vi "To Pretty String (Object).vi"(6 "pretty print? (T)":bool=TRUE, 7 "enable LabVIEW extensions? (T)":bool=TRUE, 8 "error in (no error)":errorcluster, 11 "JSON Value in":refnum<class "JSON Value.lvclass">) -> (0 "error out":errorcluster, 3 "Pretty Print String":string)   [LabVIEW 2016, in "JSON Value.lvclass"]
doc: "Pretty prints the given JSON data in an easier to read format."
uses:
  JSON Value.lvclass
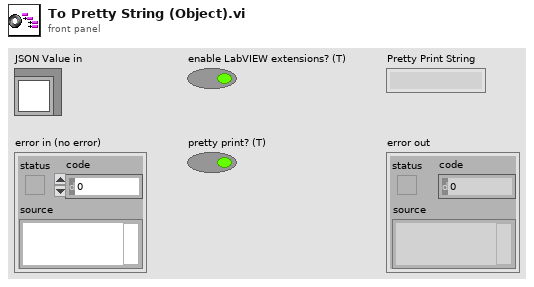
[diagram p1: front panel]
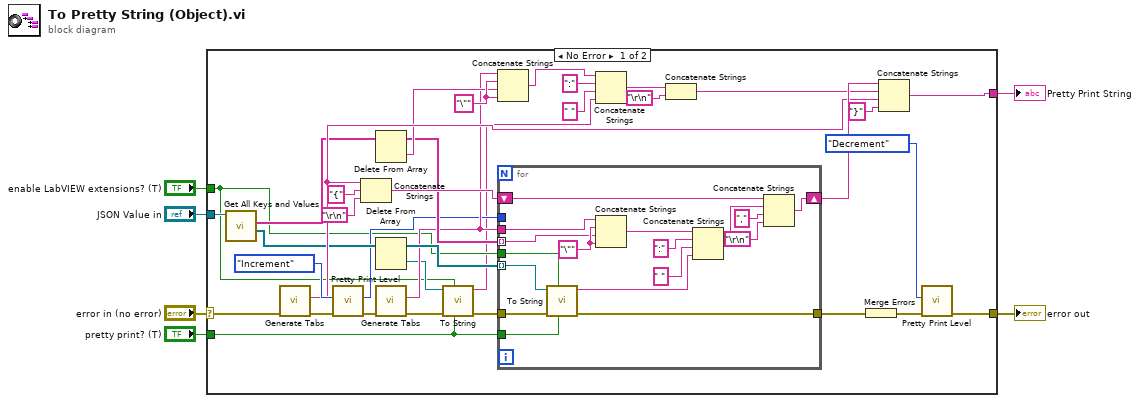
[diagram p0: block diagram]
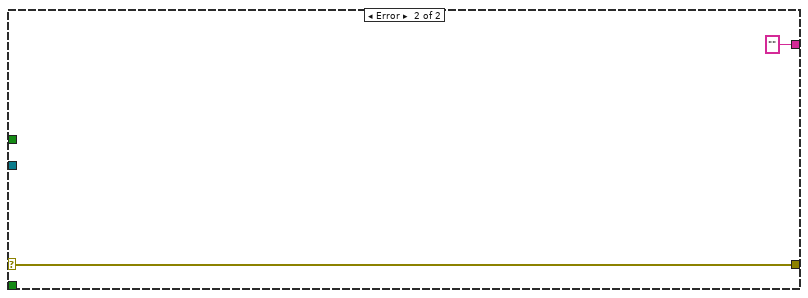
[diagram p2: hidden frame]
diagram:
  n1 = case shown="No Error" "error in (no error)" {
    selector: "error in (no error)" -> [w26 w60]
    tunnel: [w28 ""] -> w6
    tunnel: [w27 w60] -> w5
    tunnel: "JSON Value in" -> [w17 _]
    tunnel: "enable LabVIEW extensions? (T)" -> [w9 _]
    tunnel: "pretty print? (T)" -> [w8 _]
    frame No Error {
      w22 = "\"" ("string")
      n2 = call "Get All Keys and Values.vi"("JSON Value in"=w17) -> ("values"=w25:refnum<class "JSON Value.lvclass">[], "keys"=w24:string[])  [unwired: 8 in, 1 out]
      n3 = call "Generate Tabs.vi"("error in (no error)"=w26) -> ("error out"=w39:errorcluster, "Tabs"=w29:string)  [unwired: 9 in]
      n4 = call "Pretty Print Level.vi"("error in (no error)"=w39, "Action"=enum16{"Increment", "Decrement", "Get", "Reset"}."Increment") -> ("error out"=w36:errorcluster, "Numeric"=w10:i32)  [unwired: 8 in]
      n5 = Concatenate Strings(w29, "{" ("string"), "\r\n") -> (w40:string)
      n6 = Delete From Array(array=w24) -> (deleted portion=w20:string, array with subset deleted=w18:string[])  [unwired: 2 in]
      n7 = Delete From Array(array=w25) -> (deleted portion=w13:refnum<class "JSON Value.lvclass">, array with subset deleted=w35:refnum<class "JSON Value.lvclass">[])  [unwired: 2 in]
      n8 = call "Generate Tabs.vi"("error in (no error)"=w36) -> ("error out"=w12:errorcluster, "Tabs"=w15:string)  [unwired: 9 in]
      n9 = call "To String.vi"("pretty print? (T)"=w8, "enable LabVIEW extensions? (T)"=w9, "error in (no error)"=w12, "JSON Value in"=w13) -> ("error out"=w11:errorcluster, "String"=w7:string)  [unwired: 6 in]
      n10 = Concatenate Strings(w15, w22, w20, w22) -> (w21:string)
      n11 = for {
        tunnel: w35 -> [w47] mode=indexing
        shift-right: [w57] -> w33
        shift-left: w40 -> [w56]
        tunnel: w15 -> [w49]
        tunnel: w18 -> [w52] mode=indexing
        tunnel: w11 -> [w48]
        tunnel: [w46] -> w14
        tunnel: w10 -> [_]
        tunnel: w9 -> [w45]
        tunnel: w8 -> [w44]
        w54 = "\"" ("string")
        n12 = call "To String.vi"("pretty print? (T)"=w44, "enable LabVIEW extensions? (T)"=w45, "error in (no error)"=w48, "JSON Value in"=w47) -> ("error out"=w46:errorcluster, "String"=w43:string)  [unwired: 6 in]
        n13 = Concatenate Strings(w49, w54, w52, w54) -> (w55:string)
        n14 = Concatenate Strings(w55, ":" ("string"), " " ("string"), w43) -> (w51:string)
        n15 = Concatenate Strings(w56, w51, "," ("string"), "\r\n") -> (w57:string)
      }
      n16 = Concatenate Strings(w21, ":" ("string"), " " ("string"), w7) -> (w19:string)
      n17 = Concatenate Strings(w19, "\r\n") -> (w32:string)
      n18 = Merge Errors(w14) -> (w38:errorcluster)
      n19 = Concatenate Strings(w33, w32, w29, "}" ("string")) -> (w28:string)
      n20 = call "Pretty Print Level.vi"("error in (no error)"=w38, "Action"=enum16{"Increment", "Decrement", "Get", "Reset"}."Decrement") -> ("error out"=w27:errorcluster)  [unwired: 8 in, 1 out]
    }
    frame Error {
    }
  }
  "error out" <- w5
  "Pretty Print String" <- w6
